vi "小三轮的 Split HDC Bank1 DIO.vi"(0 "IN 7:0":u8 format="%08b") -> (1 "OUT 3:0":fxp<+,4,4> format="%04b", 2 "OUT 4":bool, 3 "OUT 7:5":fxp<+,3,3> format="%03b")   [LabVIEW 2017]
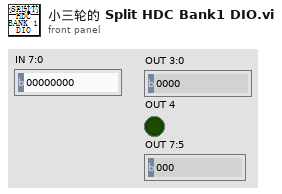
[diagram p1: front panel]
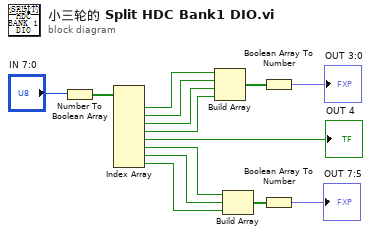
[diagram p0: block diagram]
diagram:
  n1 = Number To Boolean Array(number="IN 7:0") -> (Boolean array=w13:bool[])
  n2 = Index Array(array=w13) -> (element #1=w12:bool, element #2=w11:bool, element #3=w10:bool, element #4=w9:bool, element #5=→"OUT 4":bool, element #6=w6:bool, element #7=w5:bool, element #8=w4:bool)  [unwired: 8 in]
  n3 = Build Array(w12, w11, w10, w9) -> (w8:bool[])
  n4 = Build Array(w6, w5, w4) -> (w3:bool[])
  n5 = Boolean Array To Number(Boolean array=w8) -> (number=→"OUT 3:0":fxp<+,4,4>)
  n6 = Boolean Array To Number(Boolean array=w3) -> (number=→"OUT 7:5":fxp<+,3,3>)
